vi "Open ProviderVI.vi"(6 "password (\"\")":string, 7 "type specifier VI Refnum (for type only)":refnum<vi>, 8 "error in (no error)":errorcluster, 9 "Open Clone Reference?(F)":bool, 10 "vi path":path, 11 "application reference (local)":refnum<vi>) -> (0 "error out":errorcluster, 3 "vi reference":refnum<vi>)   [LabVIEW 2019, in "LabVIEW-ProviderShell.lvlib" / "LvProviderShellHelper.lvclass"]
uses:
  LvProviderShellHelper.lvclass
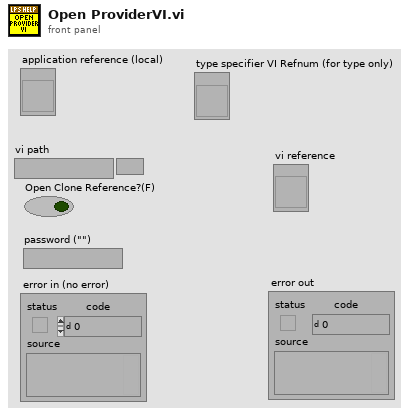
[diagram p1: front panel]
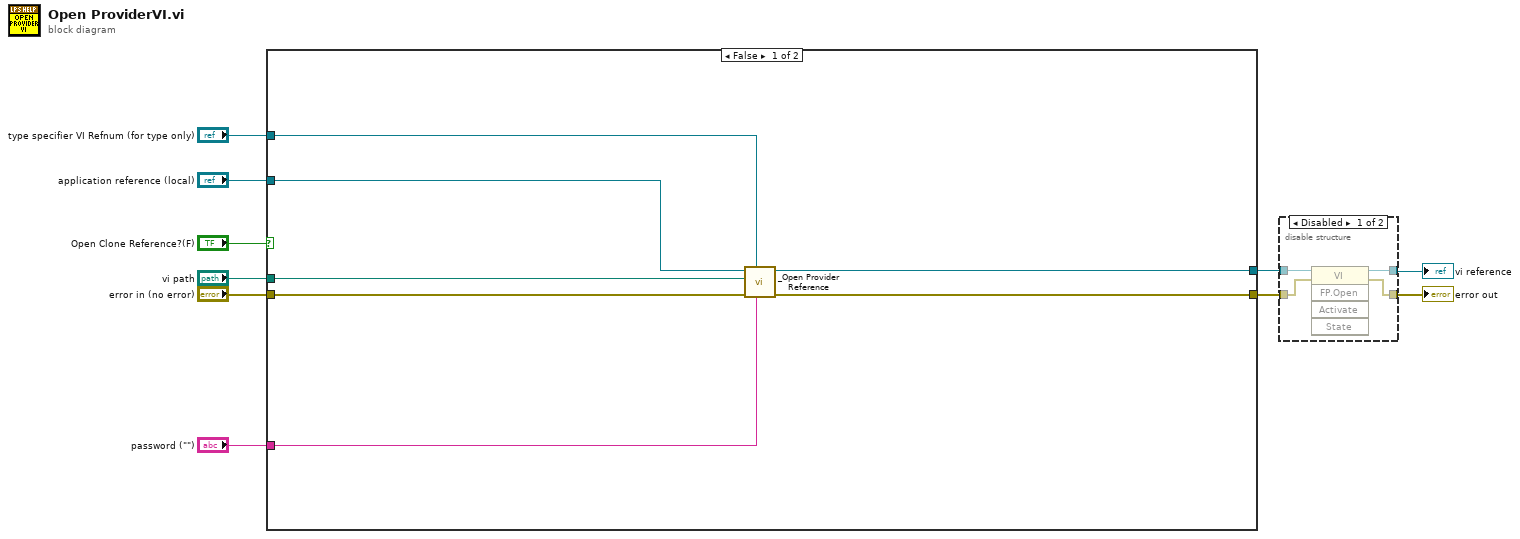
[diagram p0: block diagram]
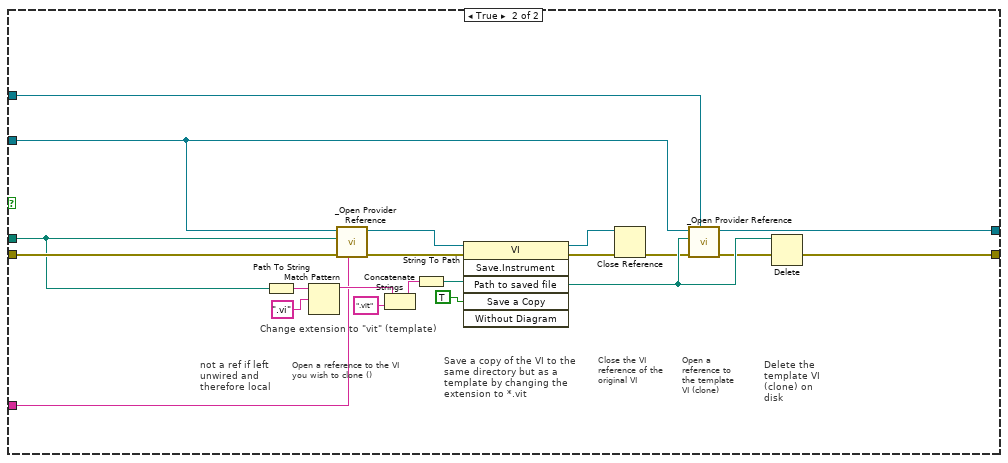
[diagram p2: hidden frame]
diagram:
  n1 = case shown="False" "Open Clone Reference?(F)" {
    tunnel: "vi path" -> [w11 w20]
    tunnel: [w17 w21] -> w10
    tunnel: [w16 w22] -> w9
    tunnel: "error in (no error)" -> [w15 w24]
    tunnel: "password (\"\")" -> [w14 w23]
    tunnel: "application reference (local)" -> [w12 w18]
    tunnel: "type specifier VI Refnum (for type only)" -> [w13 w19]
    frame False {
      n2 = call "_Open Provider Reference.vi"("password"=w14, "type specifier VI Refnum"=w13, "error in (no error)"=w15, "vi path"=w11, "application reference"=w12) -> ("error out"=w16:errorcluster, "VI out"=w17:refnum<vi>)  [unwired: 5 in]
    }
    frame True {
      # "Change extension to \"vit\" (template)"
      # "not a ref if left unwired and therefore local"
      # "Delete the template VI (clone) on disk"
      # "Open a reference to the template VI (clone)"
      # "Close the VI reference of the original VI"
      # "Save a copy of the VI to the same directory but as a template by changing the extension to *.vit"
      # "Open a reference to the VI you wish to clone ()"
      n3 = Path To String(path=w20) -> (string=w28:string)
      n4 = Match Pattern(string=w28, regular expression=".vi") -> (before substring=w29:string)  [unwired: 1 in, 3 out]
      n5 = call "_Open Provider Reference.vi"("password"=w23, "error in (no error)"=w24, "vi path"=w20, "application reference"=w18) -> ("error out"=w37:errorcluster, "VI out"=w36:refnum<vi>)  [unwired: 6 in]
      n6 = Concatenate Strings(w29, ".vit" ("regular expression")) -> (w30:string)
      n7 = String To Path(string=w30) -> (path=w35:path)
      n8 = invoke class="VI" method="Save.Instrument"(reference=w36, error in=w37, "Path to saved file"=w35, "Save a Copy"=TRUE) -> (reference out=w31:refnum<vi>, error out=w32:errorcluster)  [unwired: 2 in, 4 out]
      n9 = Close Reference(reference=w31, error in (no error)=w32) -> (error out=w33:errorcluster)
      n10 = call "_Open Provider Reference.vi"("type specifier VI Refnum"=w19, "error in (no error)"=w33, "vi path"=w35, "application reference"=w18) -> ("error out"=w34:errorcluster, "VI out"=w21:refnum<vi>)  [unwired: 6 in]
      n11 = Delete(path (use dialog)=w35, error in=w34) -> (error out=w22:errorcluster)  [unwired: 3 in, 2 out]
    }
  }
  n12 = disable-structure "Diagram Disable Structure" shown="Disabled" {
    disable-tunnel: w10 -> [w41 w43]
    disable-tunnel: [w40 w43] -> w5
    disable-tunnel: w9 -> [w39 w42]
    disable-tunnel: [w38 w42] -> w6
    frame Disabled {
      n13 = invoke class="VI" method="FP.Open"(reference=w41, error in=w39) -> (reference out=w40:refnum<vi>, error out=w38:errorcluster)  [unwired: 3 in, 3 out]
    }
    frame Enabled {
    }
  }
  "error out" <- w6
  "vi reference" <- w5
